vi "CreateQueueNames.vi"(8 "error in (no error)":errorcluster, 10 "QueueNames":string[](array[string])=["QMH", "Class", "SP"], 11 "ModuleAdmin In":refnum<class "ModuleAdmin.lvclass">) -> (0 "error out":errorcluster, 1 "Class Queue Name":string, 2 "QMH Queue Name":string, 3 "ModuleAdmin Out":refnum<class "ModuleAdmin.lvclass">, 4 "Measurement Acquisition  Loop Queue Name":string)   [LabVIEW 2018, in "AcPwrPlugins.lvlib"]
doc: "This VI creates a named queue."
uses:
  AcPwrPlugins.lvlib
  <userlib>/NIST/ModuleAdminLib/ModuleAdmin/ModuleAdmin.lvclass
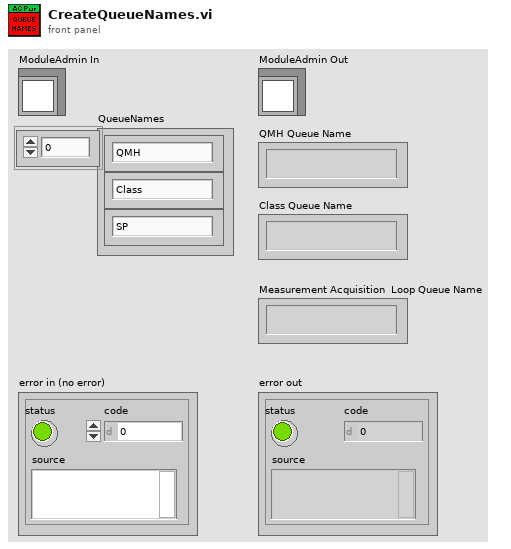
[diagram p1: front panel]
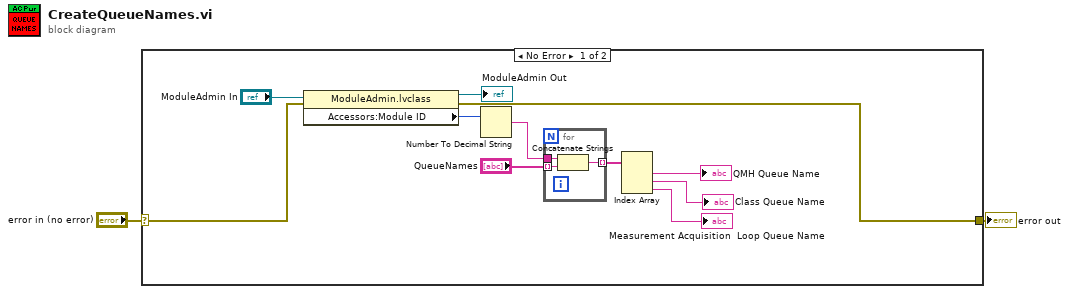
[diagram p0: block diagram]
diagram:
  n1 = case shown="No Error" "error in (no error)" {
    selector: "error in (no error)" -> [w7 w17]
    tunnel: [w5 w17] -> w2
    frame No Error {
      n2 = property class="ModuleAdmin.lvclass"(reference="ModuleAdmin In", error in=w7) -> (reference out=→"ModuleAdmin Out":refnum<class "ModuleAdmin.lvclass">, error out=w5:errorcluster, "Accessors:Module ID"=w6:i32)
      n3 = Number To Decimal String(number=w6) -> (decimal integer string=w3:string)  [unwired: 1 in]
      n4 = for {
        tunnel: [w16] -> w13 mode=indexing
        tunnel: w3 -> [w15]
        tunnel: "QueueNames" -> [w14] mode=indexing
        n5 = Concatenate Strings(w15, w14) -> (w16:string)
      }
      n6 = Index Array(array=w13) -> (element #1=→"QMH Queue Name":string, element #2=→"Class Queue Name":string, element #3=→"Measurement Acquisition  Loop Queue Name":string)  [unwired: 3 in]
    }
    frame Error {
    }
  }
  "error out" <- w2
